vi "Pump Init Selection.vi"(8 "error in (no error)":errorcluster, 11 "Pump Settings In":T1={"Output Device"=enum."Default", "Masterflex"={"VISA resource name"="", "Simulated?"=FALSE, "Pump Number"=0.0, "Reverse?"=FALSE}, "Ismatech"={"VISA resource name"="", "Simulated?"=FALSE, "Pump Number"=0.0, "Reverse?"=FALSE}, "Ismatech 3 Channel Settings"={"VISA resource name"="", "Pump Number"=1, "Channel Number"=0, "Simulated?"=TRUE, "Reverse?"=FALSE}, "VICI Settings"={"VISA resource name"="", "Pump ID"="", "Pump Head Vol"=0.0, "Reverse?"=FALSE, "Simulated?"=FALSE}, "Tacmina Settings"={"Analog DAQ Task"="", "Digital DAQ Task"=""}, "KNF SIMDOS Settings"={"VISA resource name"="", "Simulated?"=FALSE}, "ASIA Pump C"={"ASIA Pump #"=0, "channel"=0, "Simulated"=FALSE}, "FLOM Settings"={"VISA resource name"="", "Simulated?"=FALSE, "Pump Number"=0.0}, "SSI PR/LD Settings"={"VISA resource name"="", "Simulated?"=FALSE}, "SSI P40 Settings"={"VISA resource name"="", "Simulated?"=FALSE}, "Masterflex 75211 Settings"={"Analog DAQ Task"="", "Digital DAQ Task"=""}} {"Ismatech 3 Channel Settings"."Channel Number" min=0 max=3; "Ismatech 3 Channel Settings"."Pump Number" min=1; "Masterflex"."Pump Number" min=1.0 max=20.0 step=1.0; "Ismatech"."Pump Number" min=1.0 max=20.0 step=1.0; "ASIA Pump C"."channel" min=-1 max=1 step=1}) -> (0 "error out":errorcluster, 2 "Initialized":bool, 3 "Pump Settings Out":T1={"Output Device"=enum."Default", "Masterflex"={"VISA resource name"="", "Simulated?"=FALSE, "Pump Number"=0.0, "Reverse?"=FALSE}, "Ismatech"={"VISA resource name"="", "Simulated?"=FALSE, "Pump Number"=0.0, "Reverse?"=FALSE}, "Ismatech 3 Channel Settings"={"VISA resource name"="", "Pump Number"=1, "Channel Number"=0, "Simulated?"=TRUE, "Reverse?"=FALSE}, "VICI Settings"={"VISA resource name"="", "Pump ID"="", "Pump Head Vol"=0.0, "Reverse?"=FALSE, "Simulated?"=FALSE}, "Tacmina Settings"={"Analog DAQ Task"="", "Digital DAQ Task"=""}, "KNF SIMDOS Settings"={"VISA resource name"="", "Simulated?"=FALSE}, "ASIA Pump C"={"ASIA Pump #"=0, "channel"=0, "Simulated"=FALSE}, "FLOM Settings"={"VISA resource name"="", "Simulated?"=FALSE, "Pump Number"=0.0}, "SSI PR/LD Settings"={"VISA resource name"="", "Simulated?"=FALSE}, "SSI P40 Settings"={"VISA resource name"="", "Simulated?"=FALSE}, "Masterflex 75211 Settings"={"Analog DAQ Task"="", "Digital DAQ Task"=""}} {"Ismatech 3 Channel Settings"."Channel Number" min=0 max=3; "Ismatech 3 Channel Settings"."Pump Number" min=1; "Masterflex"."Pump Number" min=1.0 max=20.0 step=1.0; "Ismatech"."Pump Number" min=1.0 max=20.0 step=1.0; "ASIA Pump C"."channel" min=-1 max=1 step=1})   [LabVIEW 2018, in "Pump Module.lvlib" / "Pump Module Engine.lvlib"]
uses:
  Pump Module Engine.lvlib
  Pump Settings Cluster.ctl
  Measure Instrument/PID 2 Output Enum.ctl
  Masterflex 7550-30/Controls/Settings Cluster.ctl
  Ismatec ISM 831C/Controls/Ismatech ISM831C Settings Cluster.ctl
  Ismatec 78001/Ismatec 4083.ctl
  VICI M50 Party Mode/Settings Cluster.ctl
  Tacmina QI/Tacmina QI DAQ Setting.ctl
  KNF Pump/Settings Cluster plus SIMDOS.ctl
  ASIA Pump/Pump Settings.ctl
  FLOM Pump/Settings Cluster.ctl
  SSI PR Class/SSI PR or LD Settings Cluster.ctl
  Masterflex 75211/Masterflex 75211 DAQ Setting.ctl
  Ismatec ISM 831C/Ismatec ISM 831C.lvlib
  Masterflex 7550-30/Masterflex 7550-30.lvlib
  VICI M50 Party Mode/VICI M6 M50 Party Mode.lvlib
  Tacmina QI/Tacmina QI.lvlib
  KNF Pump/KNF SIMDOS.lvlib
  ASIA Pump.lvlib
  FLOM Pump/FLOM Pump.lvlib
  SSI PR Class/SSI PR or LD Pump.lvlib
  Masterflex 75211/Masterflex 75211.lvlib
  SSI PR Class/SSI P40 Pump.lvlib
  Ismatec 78001/Ismatec 4308.lvlib
  Pump Module.lvlib
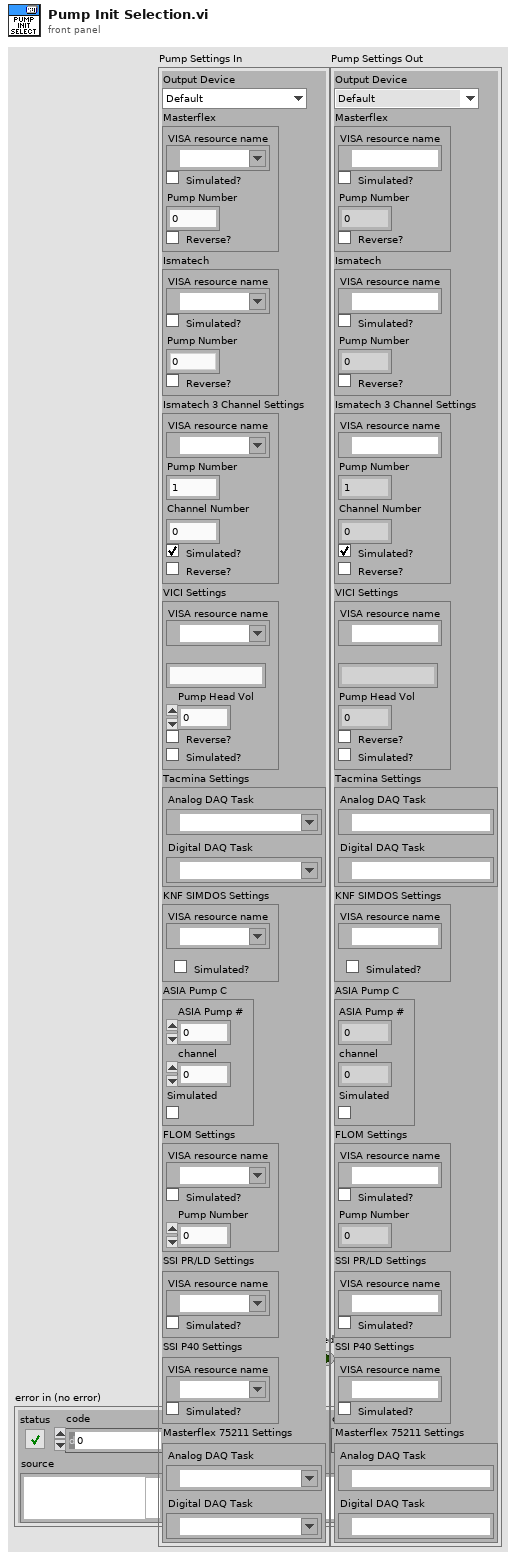
[diagram p1: front panel]
types:
  T1 = typedef "Pump Module.lvlib/Pump Settings Cluster.ctl" = cluster{"Output Device":T2, "Masterflex":T3, "Ismatech":T4, "Ismatech 3 Channel Settings":T5, "VICI Settings":T6, "Tacmina Settings":T7, "KNF SIMDOS Settings":T8, "ASIA Pump C":T9, "FLOM Settings":T10, "SSI PR/LD Settings":T11, "SSI P40 Settings":T11, "Masterflex 75211 Settings":T12}
  T2 = typedef "PID 2 Output Enum.ctl" = enum16{"Default", "Ismatec ISM 4308", "Ismatec ISM 831C", "Masterflex 7550-30", "VICI M6", "VICI M50", "Tacmina QI", "KNF SIMDOS", "ASIA Type C", "FLOM UI-22-11", "SSI PR/LD", "SSI P40", "Masterflex 75211-70"}
  T3 = typedef "Masterflex 7550-30.lvlib/Settings Cluster.ctl" = cluster{"VISA resource name":refnum<visa-resource-name>, "Simulated?":bool, "Pump Number":dbl, "Reverse?":bool}
  T4 = typedef "Ismatec ISM 831C.lvlib/Ismatech ISM831C Settings Cluster.ctl" = cluster{"VISA resource name":refnum<visa-resource-name>, "Simulated?":bool, "Pump Number":dbl, "Reverse?":bool}
  T5 = typedef "Ismatec 4308.lvlib/Ismatec 4083.ctl" = cluster{"VISA resource name":refnum<visa-resource-name>, "Pump Number":i16, "Channel Number":i16, "Simulated?":bool, "Reverse?":bool}
  T6 = typedef "VICI M6 M50 Party Mode.lvlib/Settings Cluster.ctl" = cluster{"VISA resource name":refnum<visa-resource-name>, "Pump ID":string, "Pump Head Vol":dbl, "Reverse?":bool, "Simulated?":bool}
  T7 = typedef "Tacmina QI.lvlib/Tacmina QI DAQ Setting.ctl" = cluster{"Analog DAQ Task":refnum<k21>, "Digital DAQ Task":refnum<k21>}
  T8 = typedef "KNF SIMDOS.lvlib/Settings Cluster plus SIMDOS.ctl" = cluster{"VISA resource name":refnum<visa-resource-name>, "Simulated?":bool}
  T9 = typedef "ASIA Pump.lvlib/Pump Settings.ctl" = cluster{"ASIA Pump #":i32, "channel":i32, "Simulated":bool}
  T10 = typedef "FLOM Pump.lvlib/Settings Cluster.ctl" = cluster{"VISA resource name":refnum<visa-resource-name>, "Simulated?":bool, "Pump Number":dbl}
  T11 = typedef "SSI PR or LD Pump.lvlib/SSI PR or LD Settings Cluster.ctl" = cluster{"VISA resource name":refnum<visa-resource-name>, "Simulated?":bool}
  T12 = typedef "Masterflex 75211.lvlib/Masterflex 75211 DAQ Setting.ctl" = cluster{"Analog DAQ Task":refnum<k21>, "Digital DAQ Task":refnum<k21>}
  T13 = typedef "SSI P40 Pump.lvlib/SSI P40 Settings Cluster.ctl" = cluster{"VISA resource name":refnum<visa-resource-name>, "Simulated?":bool}
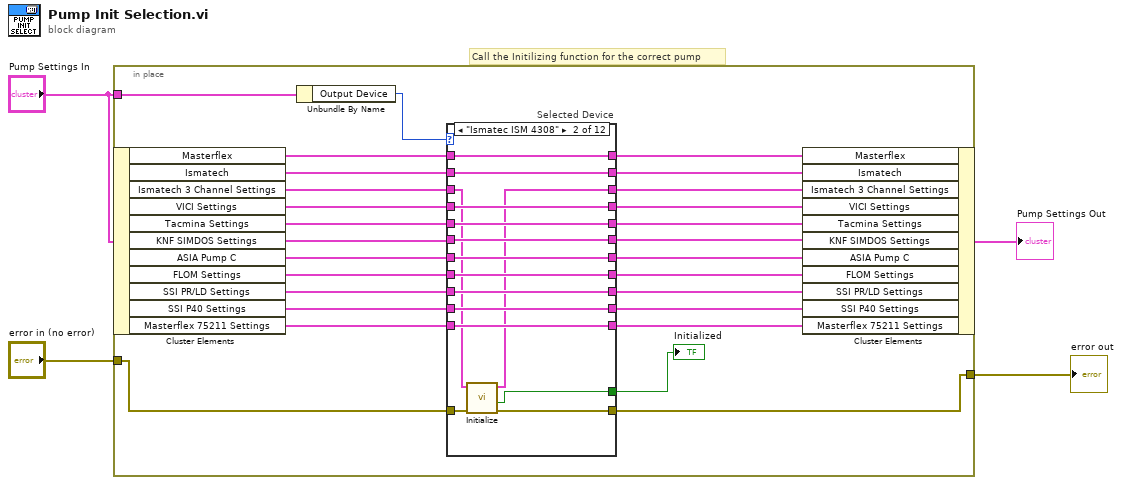
[diagram p0: block diagram]
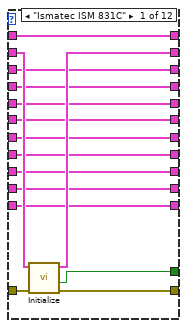
[diagram p2: hidden frame]
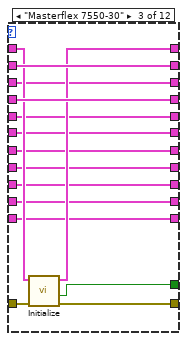
[diagram p3: hidden frame]
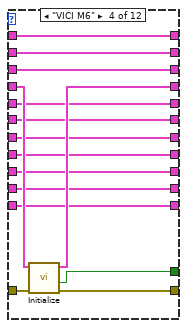
[diagram p4: hidden frame]
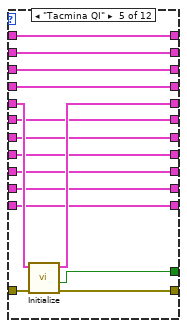
[diagram p5: hidden frame]
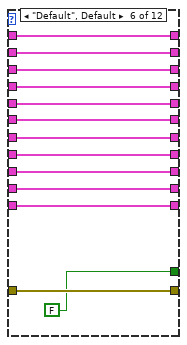
[diagram p6: hidden frame]
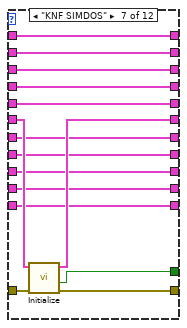
[diagram p7: hidden frame]
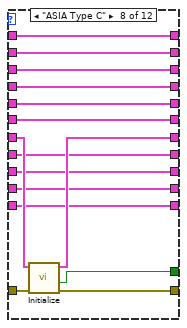
[diagram p8: hidden frame]
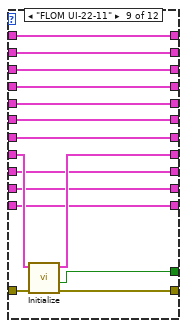
[diagram p9: hidden frame]
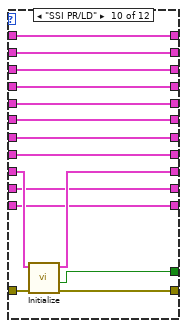
[diagram p10: hidden frame]
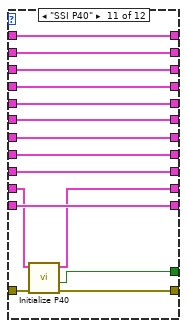
[diagram p11: hidden frame]
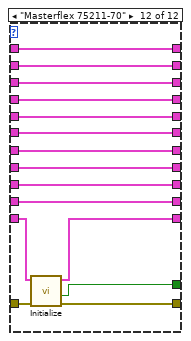
[diagram p12: hidden frame]
diagram:
  # "Call the Initilizing function for the correct pump"
  n1 = in-place {
    in-place-border: [w29] -> w4
    in-place-border: "error in (no error)" -> [w28]
    in-place-border: "Pump Settings In" -> [w27]
    n2 = in-place-cluster #1("Pump Settings In") -> ("Masterflex"=w26:T3, "Ismatech"=w25:T4, "Ismatech 3 Channel Settings"=w6:T5, "VICI Settings"=w24:T6, "Tacmina Settings"=w23:T7, "KNF SIMDOS Settings"=w22:T8, "ASIA Pump C"=w21:T9, "FLOM Settings"=w20:T10, "SSI PR/LD Settings"=w19:T11, "SSI P40 Settings"=w8:T11, "Masterflex 75211 Settings"=w9:T12)
    n3 = Unbundle By Name(w27) -> ("Output Device"=w30:T2)
    n4 = case "Selected Device" shown="\"Ismatec ISM 4308\"" w30 {
      tunnel: w26 -> [w43 w60 w74 w86 w103 w119 w134 w145 w164 w179 w194 w209]
      tunnel: [w43 w60 w73 w86 w103 w119 w134 w145 w164 w179 w194 w209] -> w18
      tunnel: w28 -> [w46 w50 w71 w88 w105 w117 w130 w149 w158 w172 w185 w201]
      tunnel: [w42 w49 w72 w89 w106 w117 w129 w148 w157 w168 w184 w200] -> w29
      tunnel: w25 -> [w45 w61 w76 w87 w104 w118 w133 w144 w163 w178 w193 w208]
      tunnel: [w44 w61 w76 w87 w104 w118 w133 w144 w163 w178 w193 w208] -> w17
      tunnel: w24 -> [w41 w59 w75 w91 w102 w116 w132 w143 w162 w177 w192 w207]
      tunnel: [w41 w59 w75 w90 w102 w116 w132 w143 w162 w177 w192 w207] -> w16
      tunnel: w23 -> [w40 w58 w70 w85 w101 w115 w131 w142 w161 w176 w191 w206]
      tunnel: [w40 w58 w70 w85 w100 w115 w131 w142 w161 w176 w191 w206] -> w15
      tunnel: w22 -> [w39 w57 w69 w84 w99 w114 w127 w141 w160 w175 w190 w205]
      tunnel: [w39 w57 w69 w84 w99 w114 w128 w141 w160 w175 w190 w205] -> w14
      tunnel: [w38 w56 w68 w83 w98 w113 w126 w147 w159 w174 w189 w204] -> w13
      tunnel: w21 -> [w38 w56 w68 w83 w98 w113 w126 w146 w159 w174 w189 w204]
      tunnel: [w37 w48 w67 w82 w97 FALSE ("Initialized") w125 w140 w156 w169 w183 w199] -> w31
      tunnel: [w36 w55 w66 w81 w96 w111 w124 w139 w155 w173 w188 w203] -> w12
      tunnel: w20 -> [w36 w55 w66 w81 w96 w111 w124 w139 w154 w173 w188 w203]
      tunnel: [w35 w54 w65 w80 w95 w110 w123 w138 w153 w170 w187 w202] -> w11
      tunnel: w19 -> [w35 w54 w65 w80 w95 w110 w123 w138 w153 w171 w187 w202]
      tunnel: [w34 w53 w64 w79 w94 w109 w122 w137 w152 w167 w186 w197] -> w10
      tunnel: w9 -> [w34 w53 w64 w79 w94 w109 w122 w137 w152 w167 w186 w198]
      tunnel: w8 -> [w33 w52 w63 w78 w93 w108 w121 w136 w151 w166 w182 w196]
      tunnel: [w33 w52 w63 w78 w93 w108 w121 w136 w151 w166 w181 w196] -> w7
      tunnel: w6 -> [w32 w51 w62 w77 w92 w107 w120 w135 w150 w165 w180 w195]
      tunnel: [w32 w47 w62 w77 w92 w107 w120 w135 w150 w165 w180 w195] -> w5
      frame "Ismatec ISM 831C" {
        n5 = call "Initialize.vi"("error in (no error)"=w46, "Ismatech Settings"=w45) -> ("error out"=w42:errorcluster, "Initialized"=w37:bool, "Ismatech Settings"=w44:T4)  [unwired: 6 in, 1 out]
      }
      frame "Ismatec ISM 4308" {
        n6 = call "Initialize.vi"("error in (no error)"=w50, "Ismatech 3 Channel Settings In"=w51) -> ("error out"=w49:errorcluster, "Initialized"=w48:bool, "Ismatech 3 Channel Settings Out"=w47:T5)  [unwired: 6 in, 1 out]
      }
      frame "Masterflex 7550-30" {
        n7 = call "Initialize.vi"("error in (no error)"=w71, "Masterflex Settings in"=w74) -> ("error out"=w72:errorcluster, "Initialized"=w67:bool, "Masterflex Settings out"=w73:T3)  [unwired: 6 in, 1 out]
      }
      frame "VICI M6" {
        n8 = call "Initialize.vi"("error in (no error)"=w88, "VICI Settings"=w91) -> ("error out"=w89:errorcluster, "Initialized"=w82:bool, "VICI Settings"=w90:T6)  [unwired: 6 in, 1 out]
      }
      frame "Tacmina QI" {
        n9 = call "Initialize.vi"("error in"=w105, "Tacmina Settings in"=w101) -> ("error out"=w106:errorcluster, "Initialized"=w97:bool, "Tacmina Settings out"=w100:T7)  [unwired: 7 in]
      }
      frame "Default", Default {
      }
      frame "KNF SIMDOS" {
        n10 = call "Initialize.vi"("error in (no error)"=w130, "KNF Settings In"=w127) -> ("error IO"=w129:errorcluster, "Initialized"=w125:bool, "KNF Settings Out"=w128:T8)  [unwired: 6 in, 1 out]
      }
      frame "ASIA Type C" {
        n11 = call "Initialize.vi"("error in (no error)"=w149, "ASIA Pump C Settings in"=w146) -> ("error out"=w148:errorcluster, "Initialized"=w140:bool, "ASIA Pump C Settings out"=w147:T9)  [unwired: 6 in, 1 out]
      }
      frame "FLOM UI-22-11" {
        n12 = call "Initialize.vi"("error in (no error)"=w158, "FLOM Settings in"=w154) -> ("error out"=w157:errorcluster, "Initialized"=w156:bool, "FLOM Settings out"=w155:T10)  [unwired: 6 in, 1 out]
      }
      frame "SSI PR/LD" {
        n13 = call "Initialize.vi"("error in (no error)"=w172, "SSI PR Settings In"=w171) -> ("error out"=w168:errorcluster, "Initialized"=w169:bool, "SSI PR Settings Out"=w170:T11)  [unwired: 6 in, 1 out]
      }
      frame "SSI P40" {
        n14 = call "Initialize P40.vi"("error in (no error)"=w185, "SSI P40 Settings In"=w182) -> ("error out"=w184:errorcluster, "Initialized"=w183:bool, "SSI P40 Settings Out"=w181:T13)  [unwired: 6 in, 1 out]
      }
      frame "Masterflex 75211-70" {
        n15 = call "Initialize.vi"("error in"=w201, "Masterflex 75211 Settings"=w198) -> ("error out"=w200:errorcluster, "Initialized"=w199:bool, "Masterflex 75211 Settings"=w197:T12)  [unwired: 7 in]
      }
    }
    "Initialized" <- w31
    n16 = in-place-cluster #1("Masterflex"=w18, "Ismatech"=w17, "Ismatech 3 Channel Settings"=w5, "VICI Settings"=w16, "Tacmina Settings"=w15, "KNF SIMDOS Settings"=w14, "ASIA Pump C"=w13, "FLOM Settings"=w12, "SSI PR/LD Settings"=w11, "SSI P40 Settings"=w7, "Masterflex 75211 Settings"=w10) -> (→"Pump Settings Out":T1)
  }
  "error out" <- w4
